vi "Spaceship_FGV.vi"(7 "Spaceship_mods":T3, 8 "error in":errorcluster, 11 "DataIn":variant) -> (0 "error out":errorcluster)   [LabVIEW 2017]
uses:
  Spaceship_mods.ctl
  Spaceship_data.ctl
  GameConfig/GameConfig_data.ctl
  Display/Display_mods.ctl
panel:
  out "Spaceship_data out":T1={"Angle"=0.0, "XVeloc"=0.0, "YVeloc"=0.0, "AngVeloc"=0.0, "GameConfig_data"={"SpaceShip"={"Angle"=30.0, "SideLenght"=2.0, "MaxLinearVeloc"=10.0, "MaxAngularVeloc"=10.0, "LinearAceleration"=1.0, "AngularAceleration"=1.0}, "Physics"={"LinearDragFactor"=1.0, "AngularDragFactor"=1.0}, "Asteroids"={"MaxSize"=6.0, "MaxDivisions"=3, "MaxVeloc"=8.0, "MinVeloc"=1.0, "Fill"=FALSE}, "Environment"={"MaxAsteroids"=10, "TimeIncrement"=0.1, "AsterProbCreation"=0.1}}, "Xpos"=0.0, "Ypos"=0.0, "Xmax"=0.0, "Ymax"=0.0}
  out "DataOut":variant
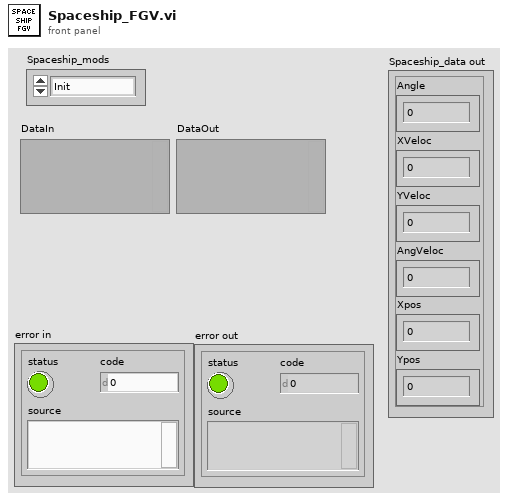
[diagram p1: front panel]
types:
  T1 = typedef "Spaceship_data.ctl" = cluster{"Angle":dbl, "XVeloc":dbl, "YVeloc":dbl, "AngVeloc":dbl, "GameConfig_data":T2, "Xpos":dbl, "Ypos":dbl, "Xmax":dbl, "Ymax":dbl}
  T2 = typedef "GameConfig_data.ctl" = cluster{"SpaceShip":cluster{"Angle":dbl, "SideLenght":dbl, "MaxLinearVeloc":dbl, "MaxAngularVeloc":dbl, "LinearAceleration":dbl, "AngularAceleration":dbl}, "Physics":cluster{"LinearDragFactor":dbl, "AngularDragFactor":dbl}, "Asteroids":cluster{"MaxSize":dbl, "MaxDivisions":i32, "MaxVeloc":dbl, "MinVeloc":dbl, "Fill":bool}, "Environment":cluster{"MaxAsteroids":i32, "TimeIncrement":dbl, "AsterProbCreation":dbl}}
  T3 = typedef "Spaceship_mods.ctl" = enum16{"Init", "Move", "Rotate", "Translate", "End"}
  T4 = typedef "Display_mods.ctl" = enum16{"Init", "GetBase", "DrawAster", "DrawShip", "Clear", "Close"}
  T5 = typedef "LVBoundsTypeDef.ctl" = cluster{"Width":u32, "Height":u32}
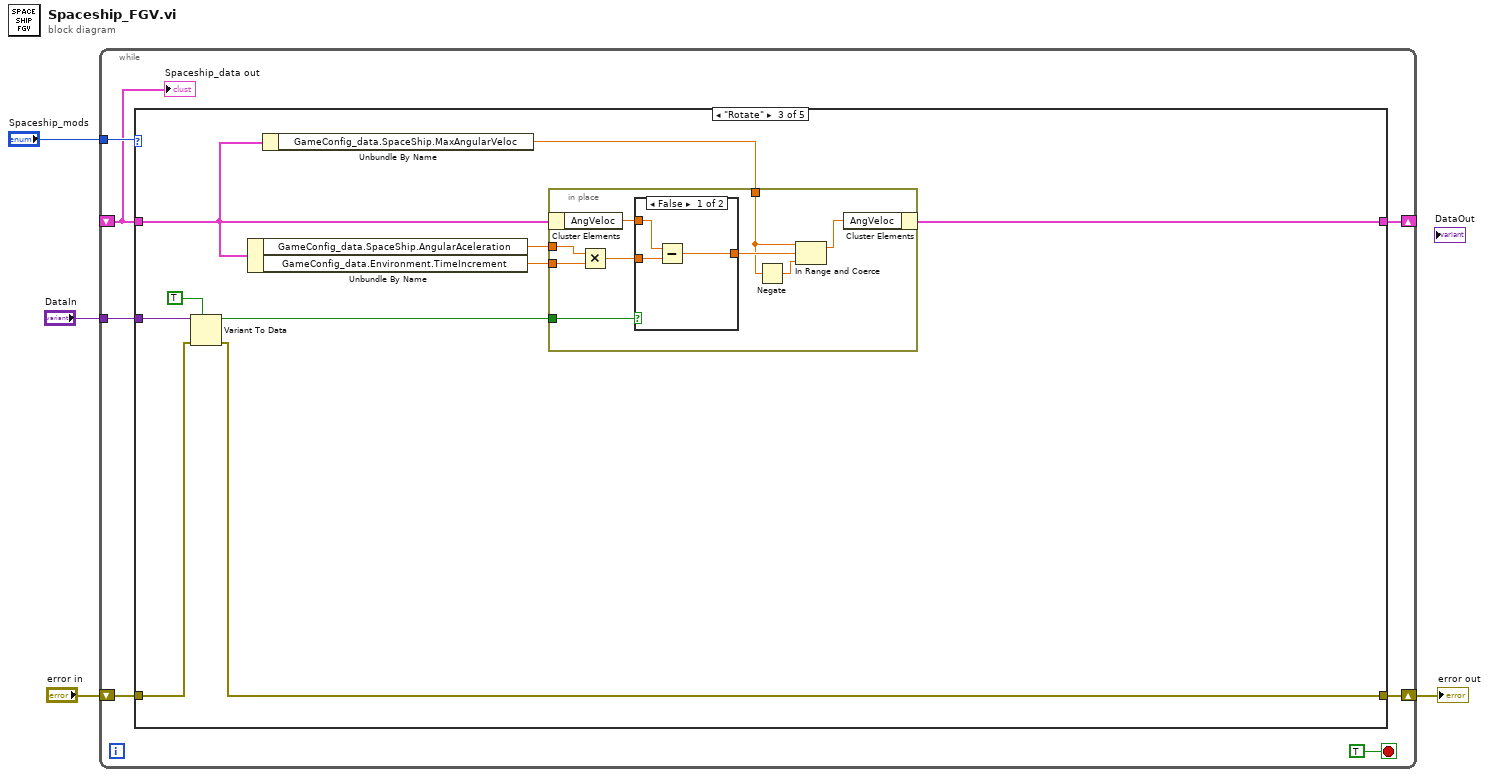
[diagram p0: block diagram]
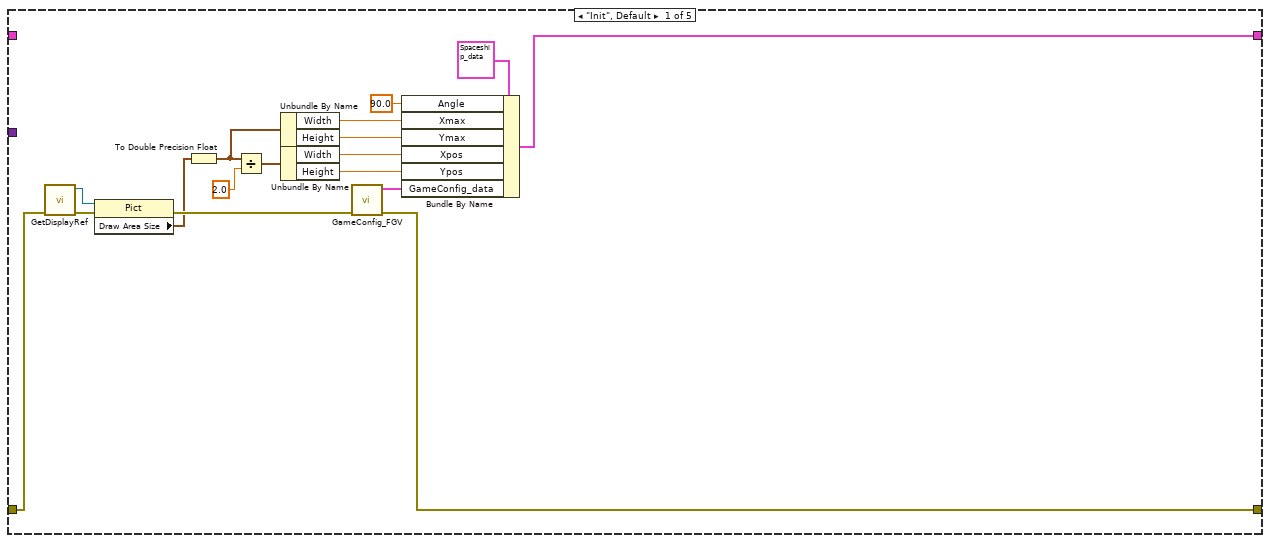
[diagram p2: hidden frame]
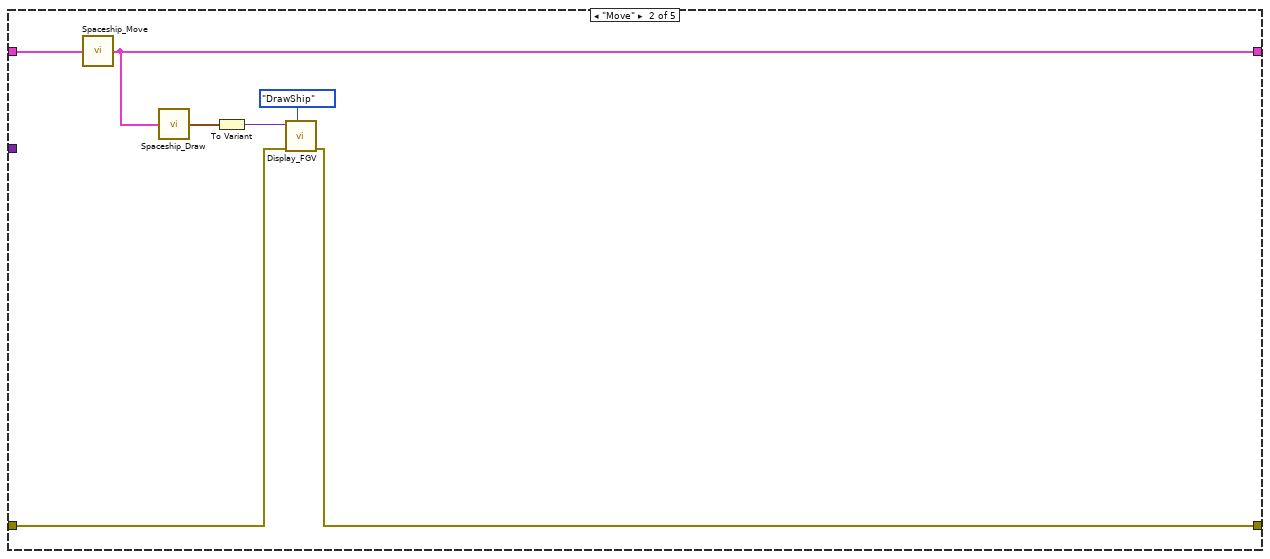
[diagram p3: hidden frame]
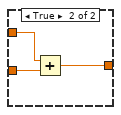
[diagram p4: hidden frame]
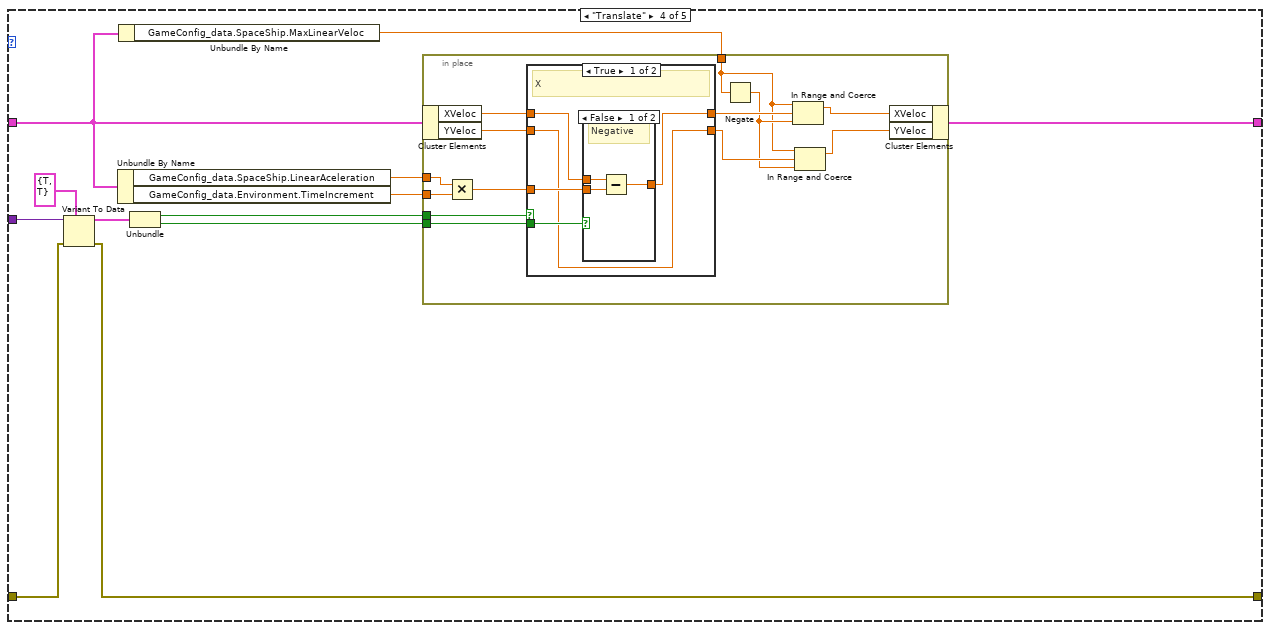
[diagram p5: hidden frame]
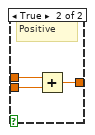
[diagram p6: hidden frame]
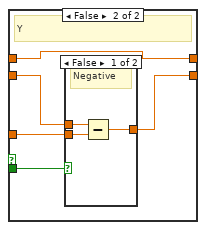
[diagram p7: hidden frame]
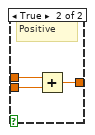
[diagram p8: hidden frame]
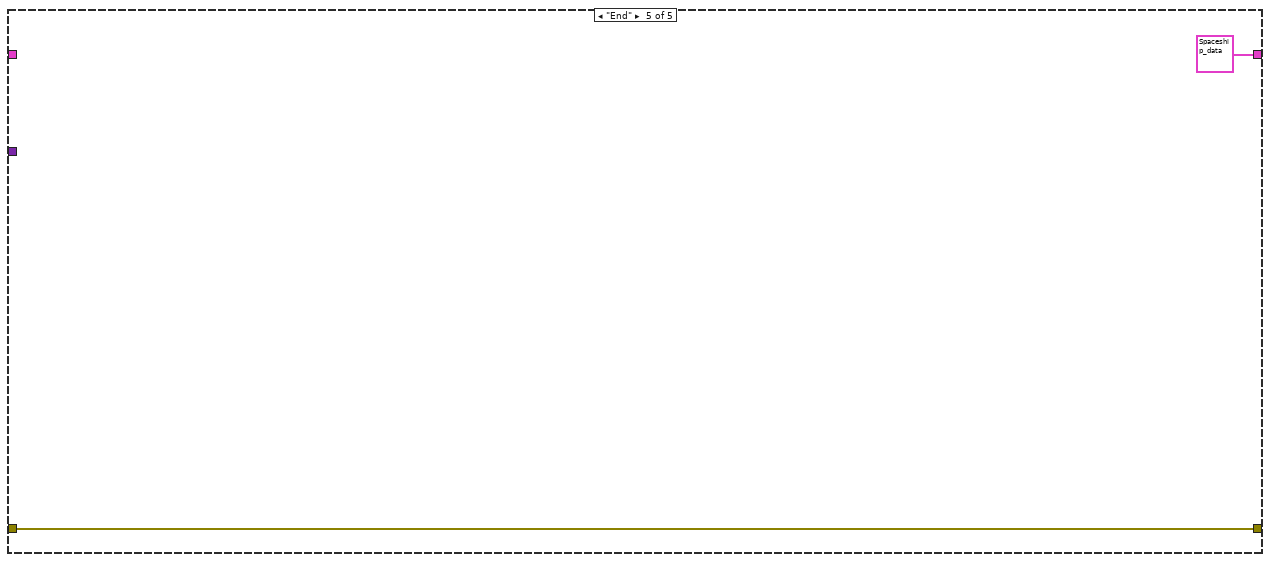
[diagram p9: hidden frame]
diagram:
  n1 = while {
    shift-right: [w7] -> w3
    shift-left: "error in" -> [w11]
    tunnel: "DataIn" -> [w9]
    tunnel: "Spaceship_mods" -> [w8]
    shift-right: [w6] -> _
    shift-left: _ -> [w5]
    stop <- TRUE stop-if-true
    n2 = case shown="\"Rotate\"" w8 {
      tunnel: w11 -> [w24 w32 w44 w71 w108]
      tunnel: w9 -> [_ _ w45 w72 _]
      tunnel: [w26 w29 w40 w68 w108] -> w7
      tunnel: [w25 w34 w38 w67 T1 {"Angle"=0.0, "XVeloc"=0.0, "YVeloc"=0.0, "AngVeloc"=0.0, "GameConfig_data"={"SpaceShip"={"Angle"=30.0, "SideLenght"=2.0, "MaxLinearVeloc"=10.0, "MaxAngularVeloc"=10.0, "LinearAceleration"=1.0, "AngularAceleration"=1.0}, "Physics"={"LinearDragFactor"=1.0, "AngularDragFactor"=1.0}, "Asteroids"={"MaxSize"=6.0, "MaxDivisions"=3, "MaxVeloc"=8.0, "MinVeloc"=1.0, "Fill"=FALSE}, "Environment"={"MaxAsteroids"=10, "TimeIncrement"=0.1, "AsterProbCreation"=0.1}}, "Xpos"=0.0, "Ypos"=0.0, "Xmax"=0.0, "Ymax"=0.0} ("Spaceship_data out")] -> w6
      tunnel: w5 -> [_ w35 w37 w66 _]
      frame "Init", Default {
        n3 = call "GetDisplayRef.vi"("error in"=w24) -> ("error out"=w20:errorcluster, "Picture out"=w23:refnum<vi>)  [unwired: 9 in]
        n4 = property class="Pict"(reference=w23, error in=w20) -> (error out=w19:errorcluster, "Draw Area Size"=w16:T5)  [unwired: 1 out]
        n5 = To Double Precision Float(number=w16) -> (double precision float=w15:cluster{"Width":dbl, "Height":dbl})
        n6 = Divide(x=w15, y=2.0) -> (x/y=w21:cluster{"Width":dbl, "Height":dbl})
        n7 = Unbundle By Name(w15) -> ("Width"=w14:dbl, "Height"=w13:dbl)
        n8 = Unbundle By Name(w21) -> ("Width"=w18:dbl, "Height"=w17:dbl)
        n9 = call "GameConfig_FGV.vi"("error in"=w19) -> ("error out"=w26:errorcluster, "Config"=w28:T2)  [unwired: 9 in]
        n10 = Bundle By Name(cluster=T1 {"Angle"=0.0, "XVeloc"=0.0, "YVeloc"=0.0, "AngVeloc"=0.0, "GameConfig_data"={"SpaceShip"={"Angle"=30.0, "SideLenght"=2.0, "MaxLinearVeloc"=10.0, "MaxAngularVeloc"=10.0, "LinearAceleration"=1.0, "AngularAceleration"=1.0}, "Physics"={"LinearDragFactor"=1.0, "AngularDragFactor"=1.0}, "Asteroids"={"MaxSize"=6.0, "MaxDivisions"=3, "MaxVeloc"=8.0, "MinVeloc"=1.0, "Fill"=FALSE}, "Environment"={"MaxAsteroids"=10, "TimeIncrement"=0.1, "AsterProbCreation"=0.1}}, "Xpos"=0.0, "Ypos"=0.0, "Xmax"=0.0, "Ymax"=0.0} ("Spaceship_data"), "Angle"=90.0, "Xmax"=w14, "Ymax"=w13, "Xpos"=w18, "Ypos"=w17, "GameConfig_data"=w28) -> (w25:T1)
      }
      frame "Move" {
        n11 = call "Spaceship_Move.vi"("Spaceship_data in"=w35) -> ("Spaceship_data out"=w34:T1)
        n12 = call "Spaceship_Draw.vi"("Spaceship_data out"=w34) -> ("SpaceshipLines"=w33:cluster{"x":i16, "y":i16}[])
        n13 = To Variant(anything=w33) -> (Variant=w30:variant)
        n14 = call "Display_FGV.vi"("Display_mods"=Display_mods."DrawShip", "error in"=w32, "variant"=w30) -> ("error out"=w29:errorcluster)  [unwired: 7 in, 1 out]
      }
      frame "Rotate" {
        n15 = Variant To Data(error in=w44, type=TRUE, Variant=w45) -> (data=w39:bool, error out=w40:errorcluster)
        n16 = Unbundle By Name(w37) -> ("GameConfig_data.SpaceShip.AngularAceleration"=w42:dbl, "GameConfig_data.Environment.TimeIncrement"=w41:dbl)
        n17 = Unbundle By Name(w37) -> ("GameConfig_data.SpaceShip.MaxAngularVeloc"=w36:dbl)
        n18 = in-place {
          in-place-border: w42 -> [w54]
          in-place-border: w41 -> [w53]
          in-place-border: w39 -> [w52]
          in-place-border: w36 -> [w47]
          n19 = in-place-cluster #1(w37) -> ("AngVeloc"=w50:dbl)
          n20 = Multiply(x=w54, y=w53) -> (x*y=w51:dbl)
          n21 = case shown="False" w52 {
            tunnel: w51 -> [w57 w60]
            tunnel: w50 -> [w56 w59]
            tunnel: [w55 w58] -> w49
            frame False {
              n22 = Subtract(x=w56, y=w57) -> (x-y=w55:dbl)
            }
            frame True {
              n23 = Add(x=w59, y=w60) -> (x+y=w58:dbl)
            }
          }
          n24 = Negate(x=w47) -> (-x=w46:dbl)
          n25 = In Range and Coerce(upper limit=w47, x=w49, lower limit=w46) -> (coerced(x)=w48:dbl)  [unwired: 1 out]
          n26 = in-place-cluster #1("AngVeloc"=w48) -> (w38:T1)
        }
      }
      frame "Translate" {
        n27 = Variant To Data(error in=w71, type=cluster{bool, bool} {TRUE, TRUE}, Variant=w72) -> (data=w65:cluster{bool, bool}, error out=w68:errorcluster)
        n28 = Unbundle By Name(w66) -> ("GameConfig_data.SpaceShip.LinearAceleration"=w70:dbl, "GameConfig_data.Environment.TimeIncrement"=w69:dbl)
        n29 = Unbundle By Name(w66) -> ("GameConfig_data.SpaceShip.MaxLinearVeloc"=w61:dbl)
        n30 = Unbundle(w65) -> (w62:bool, w63:bool)
        n31 = in-place {
          in-place-border: w70 -> [w85]
          in-place-border: w69 -> [w84]
          in-place-border: w63 -> [w81]
          in-place-border: w62 -> [w80]
          in-place-border: w61 -> [w73]
          n32 = in-place-cluster #2(w66) -> ("XVeloc"=w79:dbl, "YVeloc"=w82:dbl)
          n33 = Multiply(x=w85, y=w84) -> (x*y=w83:dbl)
          n34 = case shown="True" w80 {
            tunnel: w83 -> [w90 w101]
            tunnel: w82 -> [w86 w99]
            tunnel: w81 -> [w89 w100]
            tunnel: w79 -> [w88 w97]
            tunnel: [w87 w97] -> w78
            tunnel: [w86 w98] -> w77
            frame True {
              # "X"
              n35 = case shown="False" w89 {
                tunnel: w90 -> [w93 w96]
                tunnel: w88 -> [w92 w95]
                tunnel: [w91 w94] -> w87
                frame False {
                  # "Negative"
                  n36 = Subtract(x=w92, y=w93) -> (x-y=w91:dbl)
                }
                frame True {
                  # "Positive"
                  n37 = Add(x=w95, y=w96) -> (x+y=w94:dbl)
                }
              }
            }
            frame False {
              # "Y"
              n38 = case shown="False" w100 {
                tunnel: w101 -> [w104 w107]
                tunnel: w99 -> [w103 w106]
                tunnel: [w102 w105] -> w98
                frame False {
                  # "Negative"
                  n39 = Subtract(x=w103, y=w104) -> (x-y=w102:dbl)
                }
                frame True {
                  # "Positive"
                  n40 = Add(x=w106, y=w107) -> (x+y=w105:dbl)
                }
              }
            }
          }
          n41 = Negate(x=w73) -> (-x=w74:dbl)
          n42 = In Range and Coerce(upper limit=w73, x=w78, lower limit=w74) -> (coerced(x)=w76:dbl)  [unwired: 1 out]
          n43 = In Range and Coerce(upper limit=w73, x=w77, lower limit=w74) -> (coerced(x)=w75:dbl)  [unwired: 1 out]
          n44 = in-place-cluster #2("XVeloc"=w76, "YVeloc"=w75) -> (w67:T1)
        }
      }
      frame "End" {
      }
    }
    "Spaceship_data out" <- w5
  }
  "error out" <- w3
